vi "Hex_Cap_Convert.vi"(8 "error":errorcluster, 10 "CAP-Hex(pF)":dbl, 11 "HEX":string) -> (0 "error Out":errorcluster, 1 "Con_HEX":string, 2 "Hex-CAP (pF)":dbl, 3 "CAP(pF)":string, 4 "Con_DEC":dbl, 5 "DEC":dbl)   [LabVIEW 2012]
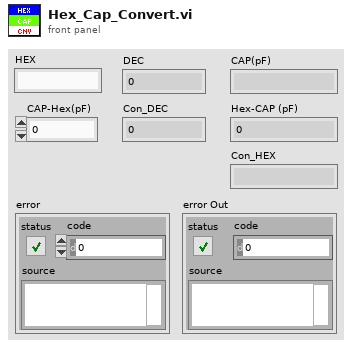
[diagram p1: front panel]
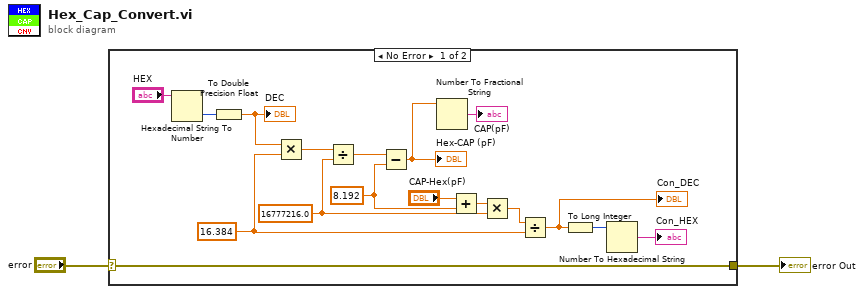
[diagram p0: block diagram]
diagram:
  n1 = case shown="No Error" "error" {
    selector: "error" -> [w3 w20]
    tunnel: [w3 w20] -> w1
    frame No Error {
      w14 = 8.192 ("y")
      w12 = 16777216.0 ("y")
      w10 = 16.384
      n2 = Hexadecimal String To Number(string="HEX") -> (number=w16:u32)  [unwired: 2 in, 1 out]
      n3 = To Double Precision Float(number=w16) -> (double precision float=w15:dbl)
      "DEC" <- w15
      n4 = Multiply(x=w15, y=w10) -> (x*y=w19:dbl)
      n5 = Divide(x=w19, y=w12) -> (x/y=w18:dbl)
      n6 = Subtract(x=w18, y=w14) -> (x-y=w6:dbl)
      "Hex-CAP (pF)" <- w6
      n7 = Number To Fractional String(number=w6) -> (F-format string=→"CAP(pF)":string)  [unwired: 3 in]
      n8 = Add(x="CAP-Hex(pF)", y=w14) -> (x+y=w13:dbl)
      n9 = Multiply(x=w13, y=w12) -> (x*y=w11:dbl)
      n10 = Divide(x=w11, y=w10) -> (x/y=w9:dbl)
      "Con_DEC" <- w9
      n11 = To Long Integer(number=w9) -> (32bit integer=w8:i32)
      n12 = Number To Hexadecimal String(2:w8) -> (0:→"Con_HEX":string)  [unwired: 1 in]
    }
    frame Error {
    }
  }
  "error Out" <- w1
